vi "Match pattern.vi"() -> ()   [LabVIEW 2011]
panel:
  out "*(type *) &x 3":string
  out "*(type *) &x 2":string
  out "*(type *) &x":string
  out "Array 2":string[](array[string])
  out "Array":string[](array[string])
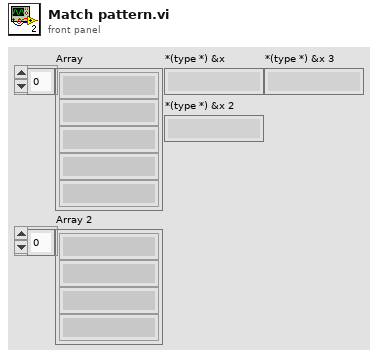
[diagram p1: front panel]
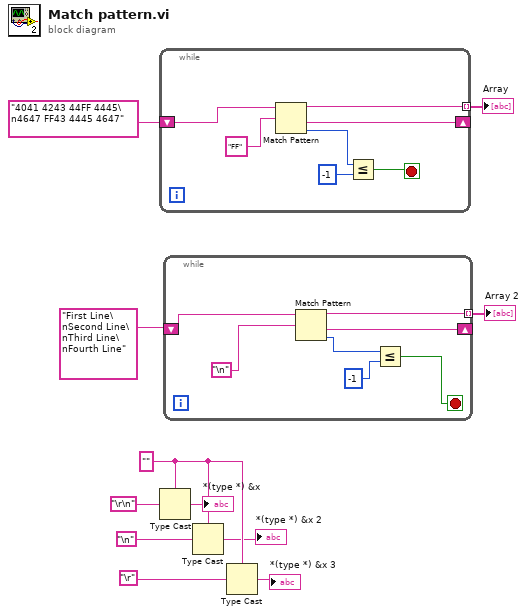
[diagram p0: block diagram]
diagram:
  w4 = "" ("type")
  n1 = while {
    tunnel: [w15] -> w10 mode=indexing
    shift-right: [w16] -> _
    shift-left: "4041 4243 44FF 4445\n4647 FF43 4445 4647" ("regular expression") -> [w17]
    stop <- w14 stop-if-true
    n2 = Match Pattern(string=w17, regular expression="FF") -> (before substring=w15:string, after substring=w16:string, offset past match=w13:i32)  [unwired: 1 in, 1 out]
    n3 = Less Or Equal?(x=w13, y=-1) -> (x <= y?=w14:bool)
  }
  "Array" <- w10
  n4 = Type Cast(type=w4, x="\r\n") -> (*(type *) &x=→"*(type *) &x":string)
  n5 = while {
    shift-right: [w24] -> _
    shift-left: "First Line\nSecond Line\nThird Line\nFourth Line" ("regular expression") -> [w25]
    tunnel: [w23] -> w8 mode=indexing
    stop <- w20 stop-if-true
    n6 = Match Pattern(string=w25, regular expression="\n") -> (before substring=w23:string, after substring=w24:string, offset past match=w22:i32)  [unwired: 1 in, 1 out]
    n7 = Less Or Equal?(x=w22, y=-1) -> (x <= y?=w20:bool)
  }
  "Array 2" <- w8
  n8 = Type Cast(type=w4, x="\n") -> (*(type *) &x=→"*(type *) &x 2":string)
  n9 = Type Cast(type=w4, x="\r") -> (*(type *) &x=→"*(type *) &x 3":string)
